vi "Trans_FPGA.vi"() -> ()   [LabVIEW 2016]
uses:
  <vilib>/LabVIEW Targets/FPGA/cRIO/shared/nicrio_ModuleControls/nicrio_cRIO-9871_BaudRateEnum.ctl
  <vilib>/LabVIEW Targets/FPGA/cRIO/shared/nicrio_ModuleControls/nicrio_cRIO-9871_ParityEnum.ctl
  <vilib>/LabVIEW Targets/FPGA/cRIO/shared/nicrio_ModuleControls/nicrio_cRIO-9871_StopBitsEnum.ctl
  <vilib>/LabVIEW Targets/FPGA/cRIO/shared/nicrio_ModuleControls/nicrio_cRIO-9871_DataBitsEnum.ctl
  <vilib>/Platform/TimedLoop/XDataNode/timing_clust.ctl
  <vilib>/Platform/TimedLoop/XDataNode/nitl_modes.ctl
  <vilib>/Platform/TimedLoop/XDataNode/wakeup.ctl
  <vilib>/rvi/FXPMathLib/basic elements/FxpIntAccumulator/subVIs/nifxpmath_IntAccumulator_SimConfig.ctl
  <vilib>/rvi/Emulation/niFpgaGetClockAttributes.vi
  <vilib>/rvi/Emulation/niFpgaSctlEmulationGetInTimedLoop.vi
  <vilib>/rvi/Emulation/niFpgaEmulationReportErrorSimple.vi
  <vilib>/rvi/eio/common/nirviEmuTemplateMethod_errors.vi
  <vilib>/rvi/Emulation/niFpgaCriticalErrorInLSC.vi
  <vilib>/rvi/Analysis/common/codeGenErrors/XNode/niFpgaXNodeCodeGenErrorHandle.vi
  <vilib>/rvi/FXPMathLib/basic elements/FxpIntAccumulator/simVIs/DllFxpIntAccumulator_sub.vi
  <vilib>/rvi/eio/common/nirviEmuTemplatePropertySet_errors.vi
  <vilib>/eio/EIONode/EIONode.xnode
  <vilib>/rvi/Analysis/measure/dc-rms/XNode/niFpgaDC-RMS.xnode
  <vilib>/Platform/TimedLoop/XDataNode/XDataNode.xnode
  <vilib>/rvi/FXPMathLib/basic elements/FxpIntAccumulator/XNode/nifxpmath_IntAccumulator.xnode
  <vilib>/rvi/FXPMathLib/FxpMul/XNode/nifxpmath_Multiplier.xnode
  <vilib>/eio/EIOPropertyNode/EIOPropertyNode.xnode
  <vilib>/eio/EIOMethodNode/EIOMethodNode.xnode
  <vilib>/Platform/TimedLoop/XDataNode/XDNodeRunTimeDep.lvlib
  <vilib>/rvi/FXPMathLib/sim/FxpSim.dll
  <vilib>/rvi/eio/common/nirviEmuTemplatePropertyGet_errors.vi
  <vilib>/rvi/eio/common/nirviEmuTemplatePropertyGet_noerrors.vi
  <vilib>/rvi/eio/common/nirviEmuTemplatePropertySet_noerrors.vi
panel:
  in  "Y-steerer+ V set":fxp<+/-,20,5>
  in  "Y-steerer- V set":fxp<+/-,20,5>
  in  "ExB+ V set":fxp<+/-,20,5>
  in  "ExB- V set":fxp<+/-,20,5>
  in  "X-steerer- V set":fxp<+/-,20,5>
  in  "X-steerer+ V set":fxp<+/-,20,5>
  out "ExB- I read":fxp<+/-,26,5>
  out "ExB- V read":fxp<+/-,26,5>
  out "ExB+ I read":fxp<+/-,26,5>
  out "ExB+ V read":fxp<+/-,26,5>
  out "Y-steerer- I read":fxp<+/-,26,5>
  out "Y-steerer- V read":fxp<+/-,26,5>
  out "Y-steerer+ I read":fxp<+/-,26,5>
  out "Y-steerer+ V read":fxp<+/-,26,5>
  out "X-steerer- I read":fxp<+/-,26,5>
  out "X-steerer- V read":fxp<+/-,26,5>
  out "X-steerer+ I read":fxp<+/-,26,5>
  out "X-steerer+ V read":fxp<+/-,26,5>
  in  "switch mag ps trig":u8[](array[numeric])=[0, 0, 0]
  in  "Switch Mag addr":u8[](array[numeric])=[0, 0, 0, 0, 0, 0, 0, 0]
  out "Switch Object Vacuum Error":errorcluster
  out "Analyze Image Vacuum Error":errorcluster
  out "Switch PS error":errorcluster
  out "ExB PS error":errorcluster
  out "Analyzer PS error":errorcluster
  out "9264 error":errorcluster
  out "9205 error":errorcluster
  in  "RT error":bool
  in  "switch mag ps set":u8[](array[numeric])=[0, 0, 0, 0, 0, 0, 0, 0, 0, 0, 0]
  out "Switch mag data":u8
  out "Switch Mag Hall Probe Timed out":bool
  out "switch mag field":u8[](array[numeric])
  out "Switch Hall Probe error":errorcluster
  in  "trans ExB mag ps set":u8[](array[numeric])=[0, 0, 0, 0, 0, 0, 0, 0, 0, 0]
  in  "analyzer mag ps set":u8[](array[numeric])=[0, 0, 0, 0, 0, 0, 0, 0, 0, 0]
  out "analyzer mag data":u8
  out "Timed Out":bool
  out "analyzer mag field":u8[](array[numeric])
  out "Analyzer Hall Probe error":errorcluster
  out "Ion gauge 4":u8[](array[numeric])
  out "Convectron 4":u8[](array[numeric])
  out "Convectron 3":u8[](array[numeric])
  out "Ion gauge 3":u8[](array[numeric])
  out "Ion gauge 2":u8[](array[numeric])
  out "Convectron 2":u8[](array[numeric])
  out "Convectron 1":u8[](array[numeric])
  out "Ion gauge 1":u8[](array[numeric])
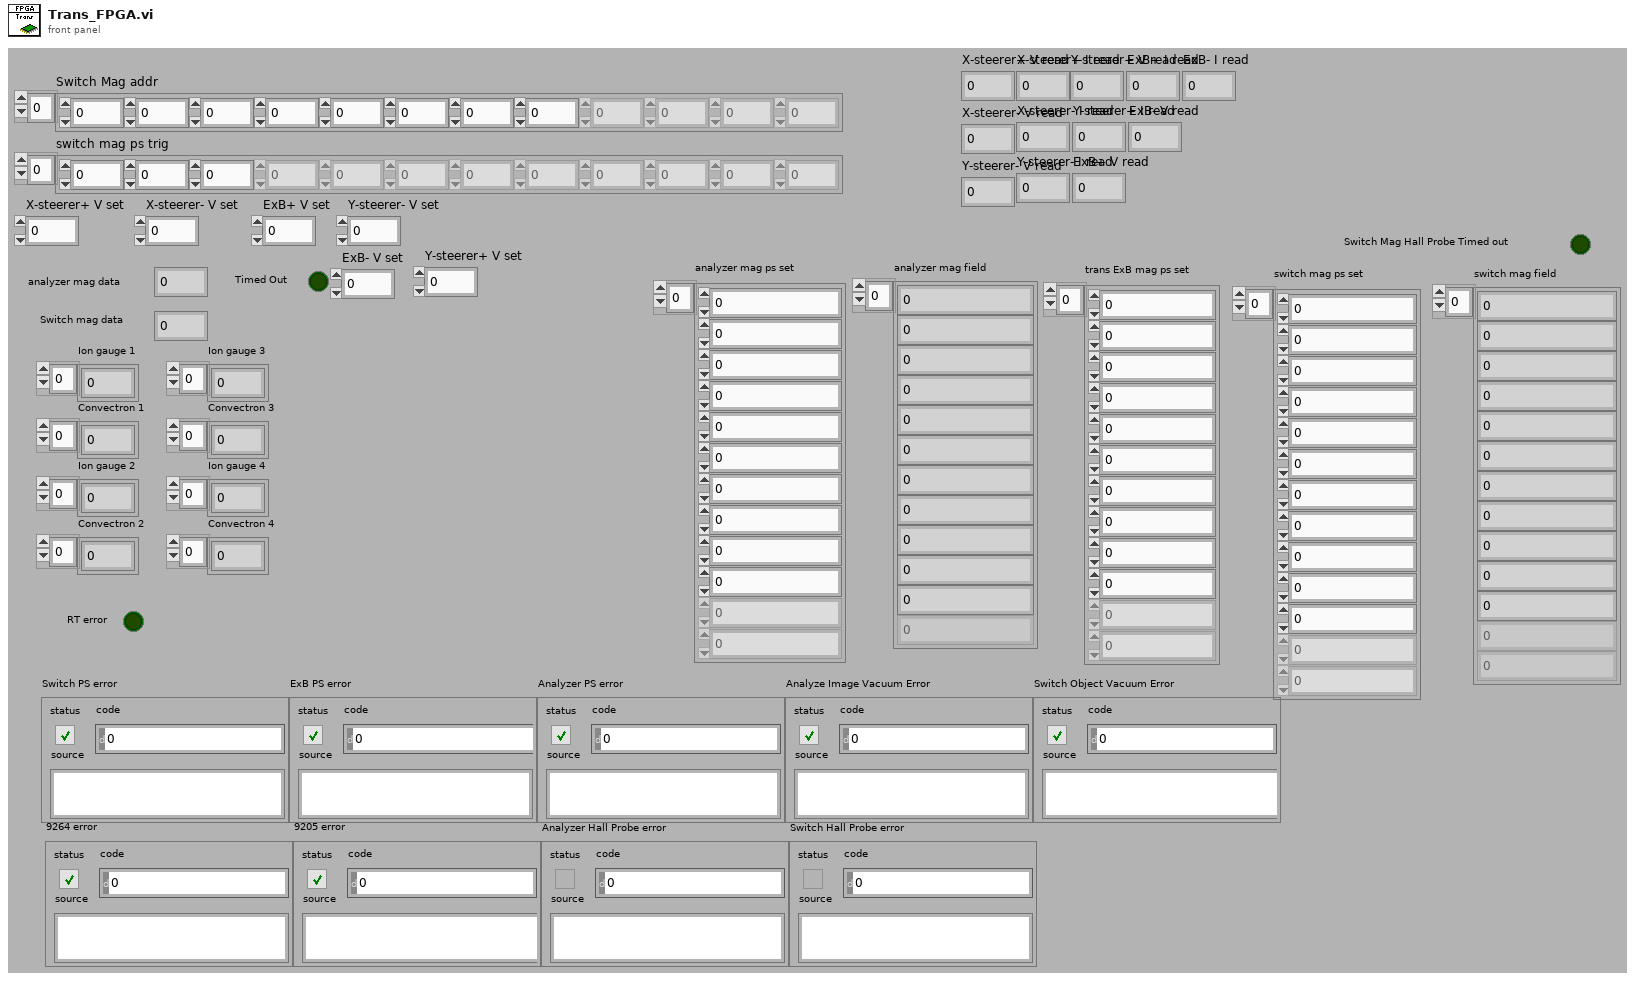
[diagram p1: front panel]
types:
  T1 = typedef "nicrio_cRIO-9871_BaudRateEnum.ctl" = enum16{"75 bps", "110 bps", "134 bps", "150 bps", "300 bps", "600 bps", "1200 bps", "1800 bps", "2400 bps", "4800 bps", "7200 bps", "9600 bps", "14.4 kbps", "19.2 kbps", "28.8 kbps", "38.4 kbps", "57.6 kbps", "115.2 kbps", "230.4 kbps", "460.8 kbps", "921.6 kbps"}
  T2 = typedef "nicrio_cRIO-9871_DataBitsEnum.ctl" = enum8{"5", "6", "7", "8"}
  T3 = typedef "nicrio_cRIO-9871_StopBitsEnum.ctl" = enum8{"1", "1.5", "2"}
  T4 = typedef "nicrio_cRIO-9871_ParityEnum.ctl" = enum8{"None", "Odd", "Even", "Mark", "Space"}
  T5 = typedef "XDNodeRunTimeDep.lvlib/timing_clust.ctl" = cluster{"Expected End [f-1]":u64, "Actual End [f-1]":u64, "Finished Late? [f-1]":bool, "Expected End [i-1]":u64, "Actual End [i-1]":u64, "Finished Late? [i-1]":bool, "Expected Start [i]":u64, "Actual Start [i]":u64, "Expected Start [f]":u64, "Actual Start [f]":u64, "Source Name":string, "Structure Name":string, "Period":i64, "Deadline":i64, "Offset":i64, "Start":i64, "Priority":i32, "Timeout":i32, "Mode":T6, "Wakeup Reason":T7, "Error":errorcluster, "Source Type":string, "Secondary Source Type":string, "Global End Time":u64, "Global Start Time":u64, "Frame Duration":u64, "Iteration Duration":u64, "Assigned CPU":i32, "I/O Scan Engine Mode":u32}
  T6 = typedef "XDNodeRunTimeDep.lvlib/nitl_modes.ctl" = enum32{"No Change", "Process missed periods, maintain original phase", "Discard missed periods, maintain original phase", "Process missed periods, ignore original phase", "Discard missed periods, ignore original phase"}
  T7 = typedef "XDNodeRunTimeDep.lvlib/wakeup.ctl" = enum32{"Normal", "Aborted", "Asynchronous wakeup", "Timing source error", "Timed loop error", "Timeout"}
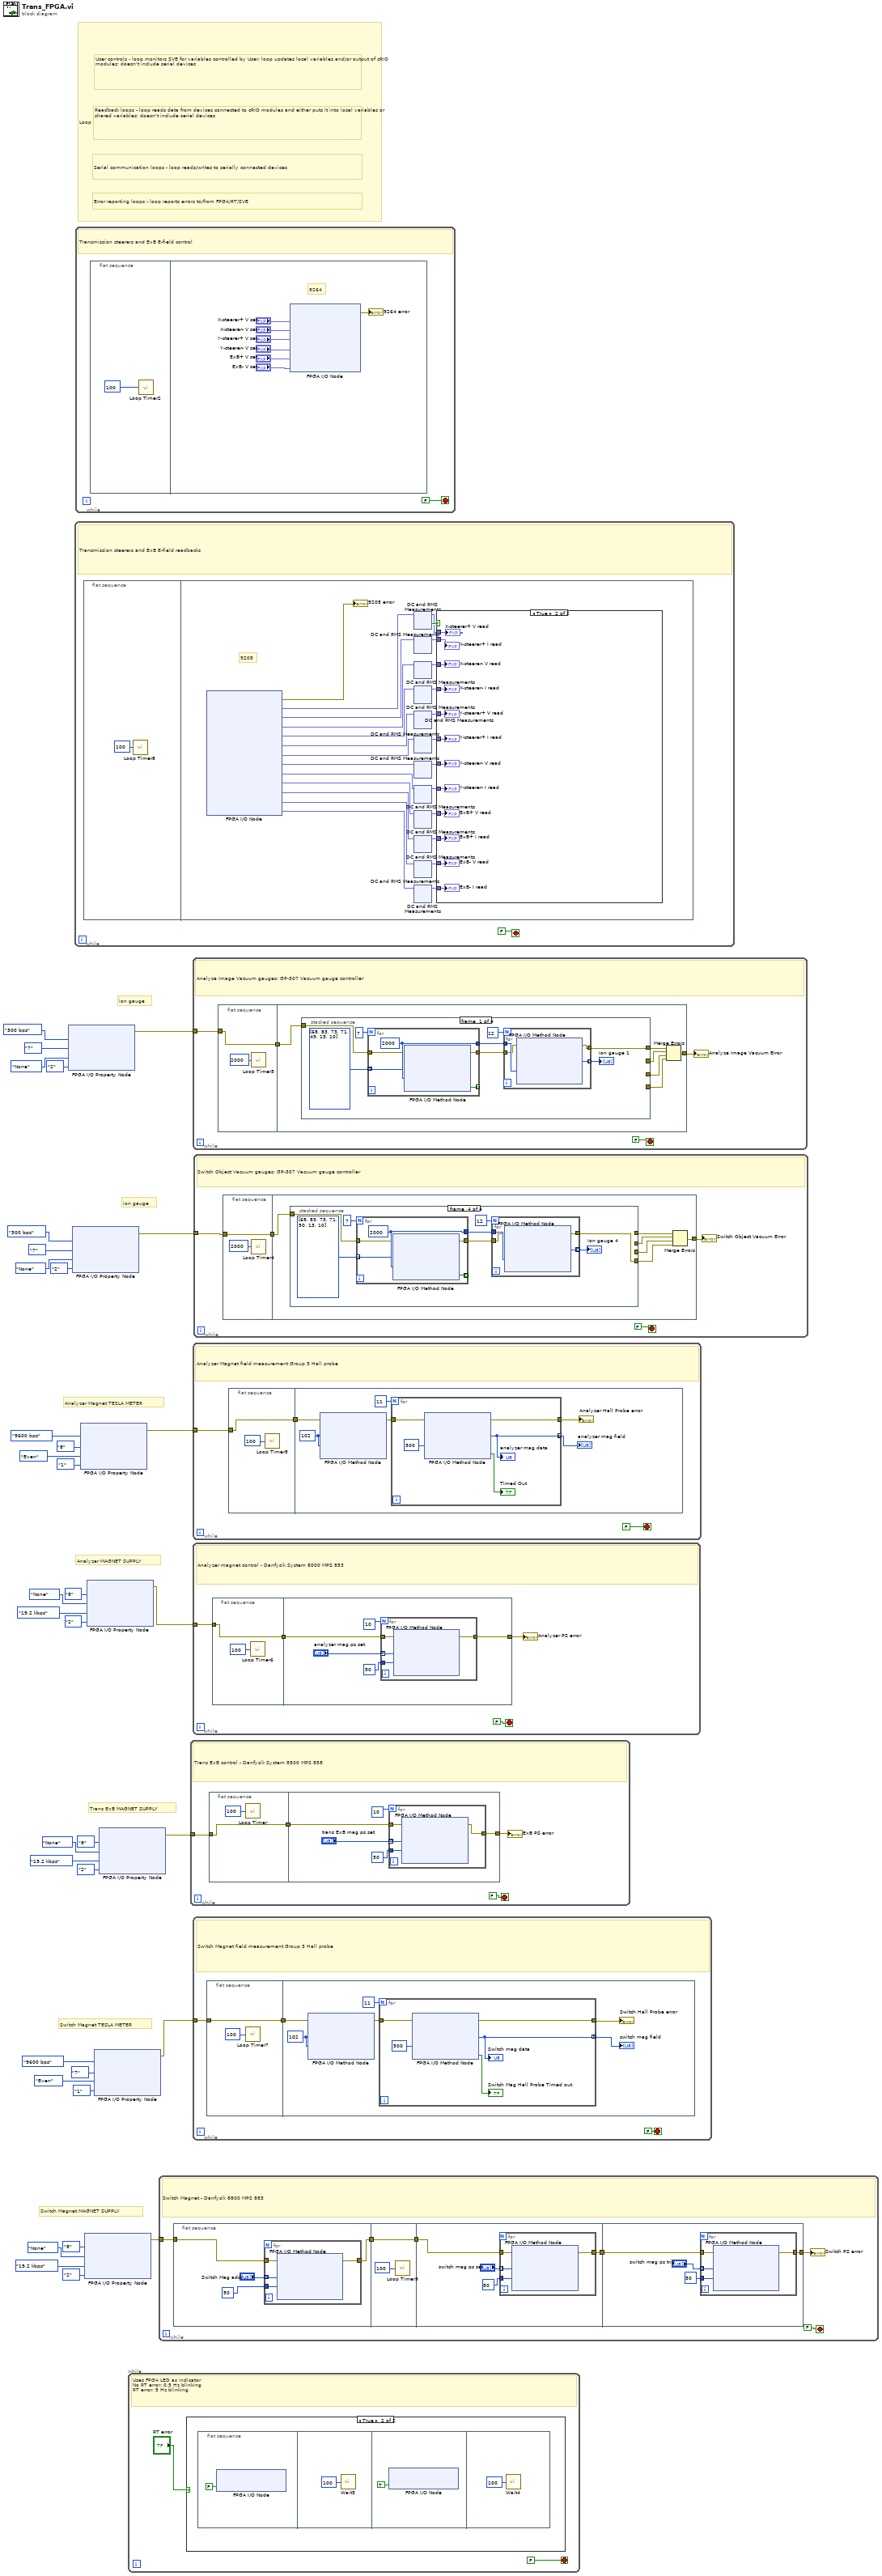
[diagram p0: block diagram]
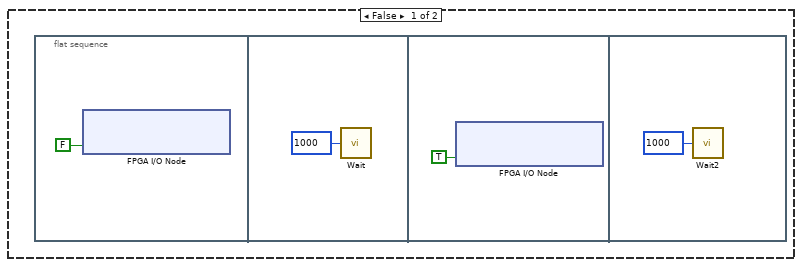
[diagram p2: hidden frame]
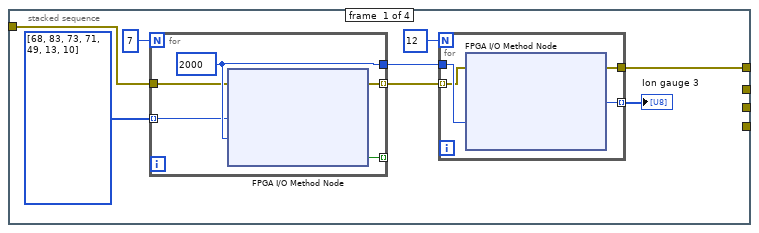
[diagram p4: hidden frame]
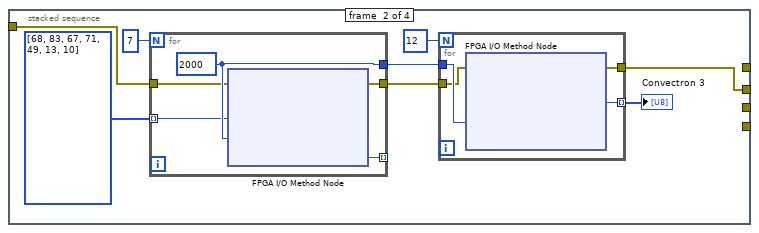
[diagram p5: hidden frame]
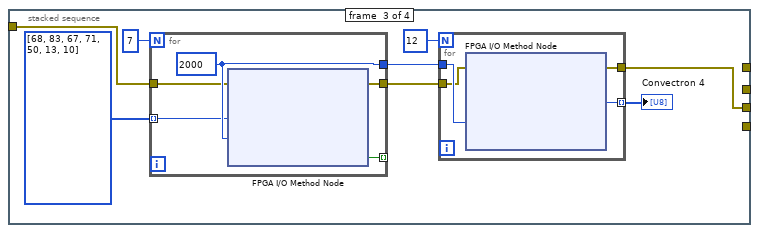
[diagram p6: hidden frame]
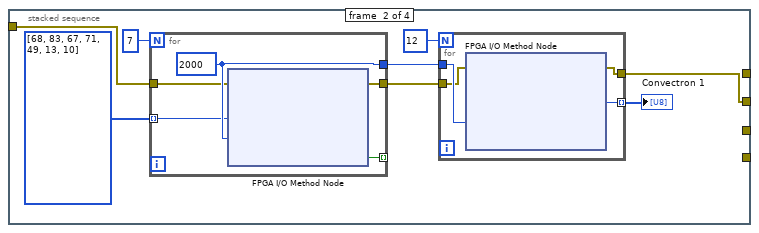
[diagram p7: hidden frame]
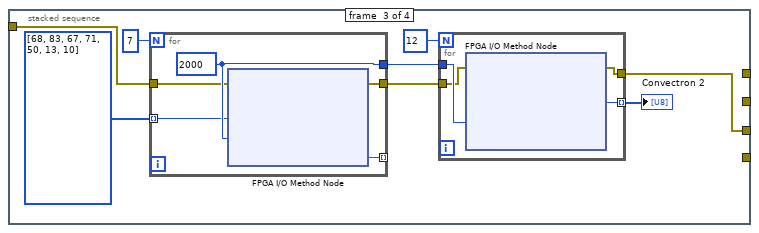
[diagram p8: hidden frame]
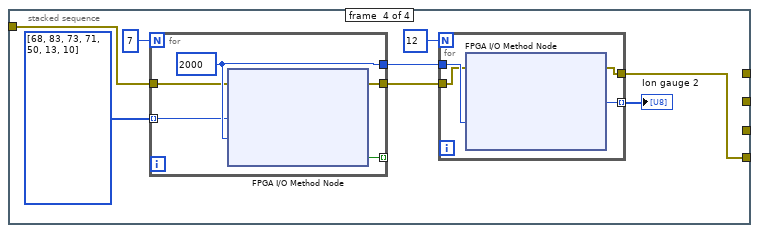
[diagram p9: hidden frame]
diagram:
  # "Error reporting loops - loop reports errors to/from FPGA/RT/SVE"
  # "Serial communication loops - loop reads/writes to serially connected devices"
  # "Readback loops - loop reads data from devices connected to cRIO modules and either puts it into local variables or shared variables; doesn't include serial devices"
  # "User controls - loop monitors SVE for variables controlled by User; loop updates local variables and/or output of cRIO modules; doesn't include serial devices"
  # "Loop legend - loops are color coded by responsibility"
  # "Switch Magnet TESLA METER"
  # "Switch Magnet MAGNET SUPPLY"
  # "Trans ExB MAGNET SUPPLY"
  # "ion gauge"
  # "Analyzer MAGNET SUPPLY"
  # "Analyzer Magnet TESLA METER"
  # "ion gauge"
  n1 = xnode "FPGA I/O Property Node"("Baud Rate"=nicrio_cRIO-9871_BaudRateEnum."300 bps", "Data Bits"=nicrio_cRIO-9871_DataBitsEnum."7", "Parity"=nicrio_cRIO-9871_ParityEnum."None", "Stop Bits"=nicrio_cRIO-9871_StopBitsEnum."2") -> ("error out"=w6:errorcluster)  [unwired: 2 in, 1 out]
  n2 = xnode "FPGA I/O Property Node"("Baud Rate"=nicrio_cRIO-9871_BaudRateEnum."300 bps", "Data Bits"=nicrio_cRIO-9871_DataBitsEnum."7", "Parity"=nicrio_cRIO-9871_ParityEnum."None", "Stop Bits"=nicrio_cRIO-9871_StopBitsEnum."2") -> ("error out"=w7:errorcluster)  [unwired: 2 in, 1 out]
  n3 = while {
    stop <- FALSE stop-if-true
    # "Transmission steerers and ExB E-field readbacks"
    n4 = flat-sequence {
      frame #0 {
        n5 = call "Loop Timer8"("Count(uSec)"=u32 100 ("Count(Ticks)")) -> ()  [unwired: 1 out]
      }
      frame #1 {
        # "9205"
        n6 = xnode "FPGA I/O Node"() -> ("error out"=→"9205 error":errorcluster, "X-steerer+ V read"=w62:fxp<+/-,26,5>, "X-steerer+ I read"=w60:fxp<+/-,26,5>, "X-steerer- V read"=w58:fxp<+/-,26,5>, "X-steerer- I read"=w56:fxp<+/-,26,5>, "Y-steerer+ V read"=w54:fxp<+/-,26,5>, "Y-steerer+ I read"=w52:fxp<+/-,26,5>, "Y-steerer- V read"=w50:fxp<+/-,26,5>, "Y-steerer- I read"=w48:fxp<+/-,26,5>, "ExB+ V read"=w46:fxp<+/-,26,5>, "ExB+ I read"=w44:fxp<+/-,26,5>, "ExB- V read"=w42:fxp<+/-,26,5>, "ExB- I read"=w40:fxp<+/-,26,5>)  [unwired: 13 in, 12 out]
        n7 = xnode "DC and RMS Measurements"("input data"=w62) -> ("DC"=w61:fxp<+/-,26,5>, "output valid"=w63:bool)  [unwired: 1 in]
        n8 = xnode "DC and RMS Measurements"("input data"=w60) -> ("DC"=w59:fxp<+/-,26,5>)  [unwired: 1 in, 1 out]
        n9 = xnode "DC and RMS Measurements"("input data"=w58) -> ("DC"=w57:fxp<+/-,26,5>)  [unwired: 1 in, 1 out]
        n10 = xnode "DC and RMS Measurements"("input data"=w56) -> ("DC"=w55:fxp<+/-,26,5>)  [unwired: 1 in, 1 out]
        n11 = xnode "DC and RMS Measurements"("input data"=w54) -> ("DC"=w53:fxp<+/-,26,5>)  [unwired: 1 in, 1 out]
        n12 = xnode "DC and RMS Measurements"("input data"=w52) -> ("DC"=w51:fxp<+/-,26,5>)  [unwired: 1 in, 1 out]
        n13 = xnode "DC and RMS Measurements"("input data"=w50) -> ("DC"=w49:fxp<+/-,26,5>)  [unwired: 1 in, 1 out]
        n14 = xnode "DC and RMS Measurements"("input data"=w48) -> ("DC"=w47:fxp<+/-,26,5>)  [unwired: 1 in, 1 out]
        n15 = xnode "DC and RMS Measurements"("input data"=w46) -> ("DC"=w45:fxp<+/-,26,5>)  [unwired: 1 in, 1 out]
        n16 = xnode "DC and RMS Measurements"("input data"=w44) -> ("DC"=w43:fxp<+/-,26,5>)  [unwired: 1 in, 1 out]
        n17 = xnode "DC and RMS Measurements"("input data"=w42) -> ("DC"=w41:fxp<+/-,26,5>)  [unwired: 1 in, 1 out]
        n18 = xnode "DC and RMS Measurements"("input data"=w40) -> ("DC"=w39:fxp<+/-,26,5>)  [unwired: 1 in, 1 out]
        n19 = case shown="True" w63 {
          tunnel: w61 -> [_ w75]
          tunnel: w59 -> [_ w74]
          tunnel: w57 -> [_ w73]
          tunnel: w55 -> [_ w72]
          tunnel: w53 -> [_ w71]
          tunnel: w51 -> [_ w70]
          tunnel: w49 -> [_ w69]
          tunnel: w47 -> [_ w68]
          tunnel: w45 -> [_ w67]
          tunnel: w43 -> [_ w66]
          tunnel: w41 -> [_ w65]
          tunnel: w39 -> [_ w64]
          frame False {
          }
          frame True {
            "X-steerer+ V read" <- w75
            "X-steerer+ I read" <- w74
            "X-steerer- V read" <- w73
            "X-steerer- I read" <- w72
            "Y-steerer+ V read" <- w71
            "Y-steerer+ I read" <- w70
            "Y-steerer- V read" <- w69
            "Y-steerer- I read" <- w68
            "ExB+ V read" <- w67
            "ExB+ I read" <- w66
            "ExB- V read" <- w65
            "ExB- I read" <- w64
          }
        }
      }
    }
  }
  n20 = while {
    stop <- FALSE stop-if-true
    # "Transmission steerers and ExB E-field control"
    n21 = flat-sequence {
      frame #0 {
        n22 = call "Loop Timer2"("Count(mSec)"=u32 100 ("Count(Ticks)")) -> ()  [unwired: 1 out]
      }
      frame #1 {
        # "9264"
        n23 = xnode "FPGA I/O Node"("X-steerer+ V set"="X-steerer+ V set", "X-steerer- V set"="X-steerer- V set", "Y-steerer+ V set"="Y-steerer+ V set", "Y-steerer- V set"="Y-steerer- V set", "ExB+ V set"="ExB+ V set", "ExB- V set"="ExB- V set") -> ("error out"=→"9264 error":errorcluster)  [unwired: 7 in, 6 out]
      }
    }
  }
  n24 = xnode "FPGA I/O Property Node"("Baud Rate"=nicrio_cRIO-9871_BaudRateEnum."9600 bps", "Data Bits"=nicrio_cRIO-9871_DataBitsEnum."8", "Parity"=nicrio_cRIO-9871_ParityEnum."Even", "Stop Bits"=nicrio_cRIO-9871_StopBitsEnum."1") -> ("error out"=w8:errorcluster)  [unwired: 2 in, 1 out]
  n25 = xnode "FPGA I/O Property Node"("Data Bits"=nicrio_cRIO-9871_DataBitsEnum."8", "Parity"=nicrio_cRIO-9871_ParityEnum."None", "Baud Rate"=nicrio_cRIO-9871_BaudRateEnum."19.2 kbps", "Stop Bits"=nicrio_cRIO-9871_StopBitsEnum."2") -> ("error out"=w10:errorcluster)  [unwired: 2 in, 1 out]
  n26 = xnode "FPGA I/O Property Node"("Data Bits"=nicrio_cRIO-9871_DataBitsEnum."8", "Parity"=nicrio_cRIO-9871_ParityEnum."None", "Baud Rate"=nicrio_cRIO-9871_BaudRateEnum."19.2 kbps", "Stop Bits"=nicrio_cRIO-9871_StopBitsEnum."2") -> ("error out"=w9:errorcluster)  [unwired: 2 in, 1 out]
  n27 = xnode "FPGA I/O Property Node"("Baud Rate"=nicrio_cRIO-9871_BaudRateEnum."9600 bps", "Data Bits"=nicrio_cRIO-9871_DataBitsEnum."7", "Parity"=nicrio_cRIO-9871_ParityEnum."Even", "Stop Bits"=nicrio_cRIO-9871_StopBitsEnum."1") -> ("error out"=w11:errorcluster)  [unwired: 2 in, 1 out]
  n28 = xnode "FPGA I/O Property Node"("Data Bits"=nicrio_cRIO-9871_DataBitsEnum."8", "Parity"=nicrio_cRIO-9871_ParityEnum."None", "Baud Rate"=nicrio_cRIO-9871_BaudRateEnum."19.2 kbps", "Stop Bits"=nicrio_cRIO-9871_StopBitsEnum."2") -> ("error out"=w12:errorcluster)  [unwired: 2 in, 1 out]
  n29 = while {
    stop <- FALSE stop-if-true
    # "Uses FPGA LED as indicator\nNo RT error: 0.5 Hz blinking\nRT error: 5 Hz blinking"
    n30 = case shown="True" "RT error" {
      frame False {
        n31 = flat-sequence {
          frame #0 {
            n32 = xnode "FPGA I/O Node"("USER FPGA LED"=FALSE ("FPGA LED")) -> ()  [unwired: 1 in, 1 out]
          }
          frame #1 {
            n33 = call "Wait"("Count(mSec)"=u16 1000) -> ()  [unwired: 1 out]
          }
          frame #2 {
            n34 = xnode "FPGA I/O Node"("USER FPGA LED"=TRUE ("FPGA LED")) -> ()  [unwired: 1 in, 1 out]
          }
          frame #3 {
            n35 = call "Wait2"("Count(mSec)"=u16 1000) -> ()  [unwired: 1 out]
          }
        }
      }
      frame True {
        n36 = flat-sequence {
          frame #0 {
            n37 = xnode "FPGA I/O Node"("USER FPGA LED"=FALSE ("FPGA LED")) -> ()  [unwired: 1 in, 1 out]
          }
          frame #1 {
            n38 = call "Wait3"("Count(mSec)"=u16 100) -> ()  [unwired: 1 out]
          }
          frame #2 {
            n39 = xnode "FPGA I/O Node"("USER FPGA LED"=TRUE ("FPGA LED")) -> ()  [unwired: 1 in, 1 out]
          }
          frame #3 {
            n40 = call "Wait4"("Count(mSec)"=u16 100) -> ()  [unwired: 1 out]
          }
        }
      }
    }
  }
  n41 = while {
    tunnel: w10 -> [w1057]
    stop <- FALSE stop-if-true
    # "Switch Magnet - Danfysik 8800 MPS 883"
    n42 = flat-sequence {
      tunnel: w1057 -> [w1063]
      tunnel: [w1062] -> w1056
      tunnel: [w1069] -> w1058
      tunnel: w1056 -> [w1069]
      tunnel: w1058 -> [w1071]
      tunnel: [w1072] -> w1055
      tunnel: [w1082] -> w1059
      tunnel: w1055 -> [w1081]
      frame #0 {
        n43 = for {
          tunnel: 50 ("Timeout (ms)") -> [w1068]
          tunnel: "Switch Mag addr" -> [w1067] mode=indexing
          tunnel: [w1066] -> w1062
          tunnel: w1063 -> [w1065]
          n44 = xnode "FPGA I/O Method Node"("error in"=w1065, "Data"=w1067, "Timeout (ms)"=w1068) -> ("error out"=w1066:errorcluster)  [unwired: 1 in, 2 out]
        }
      }
      frame #1 {
        n45 = call "Loop Timer9"("Count(mSec)"=u32 100) -> ()  [unwired: 1 out]
      }
      frame #2 {
        n46 = for {
          tunnel: 50 ("Timeout (ms)") -> [w1078]
          tunnel: "switch mag ps set" -> [w1077] mode=indexing
          tunnel: [w1076] -> w1072
          tunnel: w1071 -> [w1075]
          n47 = xnode "FPGA I/O Method Node"("error in"=w1075, "Data"=w1077, "Timeout (ms)"=w1078) -> ("error out"=w1076:errorcluster)  [unwired: 1 in, 2 out]
        }
      }
      frame #3 {
        n48 = for {
          tunnel: 50 ("Timeout (ms)") -> [w1086]
          tunnel: "switch mag ps trig" -> [w1085] mode=indexing
          tunnel: [w1084] -> w1082
          tunnel: w1081 -> [w1083]
          n49 = xnode "FPGA I/O Method Node"("error in"=w1083, "Data"=w1085, "Timeout (ms)"=w1086) -> ("error out"=w1084:errorcluster)  [unwired: 1 in, 2 out]
        }
      }
    }
    "Switch PS error" <- w1059
  }
  n50 = while {
    tunnel: w12 -> [w1088]
    stop <- FALSE stop-if-true
    # "Trans ExB control - Danfysik System 8500 MPS 858"
    n51 = flat-sequence {
      tunnel: w1088 -> [w1091]
      tunnel: [w1091] -> w1087
      tunnel: [w1094] -> w1089
      tunnel: w1087 -> [w1093]
      frame #0 {
        n52 = call "Loop Timer"("Count(mSec)"=u32 100) -> ()  [unwired: 1 out]
      }
      frame #1 {
        n53 = for {
          N: 10 -> [_]
          tunnel: 50 ("Timeout (ms)") -> [w1101]
          tunnel: "trans ExB mag ps set" -> [w1100] mode=indexing
          tunnel: [w1099] -> w1094
          tunnel: w1093 -> [w1098]
          n54 = xnode "FPGA I/O Method Node"("error in"=w1098, "Data"=w1100, "Timeout (ms)"=w1101) -> ("error out"=w1099:errorcluster)  [unwired: 1 in, 2 out]
        }
      }
    }
    "ExB PS error" <- w1089
  }
  n55 = while {
    tunnel: w6 -> [w1104]
    stop <- FALSE stop-if-true
    # "Analyze Image Vacuum gauges: GP-307 Vacuum gauge controller"
    n56 = flat-sequence {
      tunnel: w1104 -> [w1106]
      tunnel: [w1106] -> w1103
      tunnel: w1103 -> [w1113]
      tunnel: [w1111] -> w1102
      frame #0 {
        n57 = call "Loop Timer3"("Count(mSec)"=u32 2000 ("Count(Ticks)")) -> ()  [unwired: 1 out]
      }
      frame #1 {
        n58 = stacked-sequence {
          tunnel: w1113 -> [w1116 w1133 w1150 w1166]
          tunnel: [w1114 _ _ _] -> w1112
          tunnel: [_ w1131 _ _] -> w1110
          tunnel: [_ _ w1148 _] -> w1109
          tunnel: [_ _ _ w1165] -> w1108
          frame #0 {
            n59 = for {
              N: 7 -> [_]
              tunnel: [w1130] -> w1121
              tunnel: [w1129] -> _ mode=indexing
              tunnel: u8[] [68, 83, 73, 71, 49, 13, 10] ("unsigned byte array") -> [w1128] mode=indexing
              tunnel: w1116 -> [w1127]
              tunnel: [w1126] -> w1115
              w1130 = 2000 ("Timeout (ms)")
              n60 = xnode "FPGA I/O Method Node"("error in"=w1127, "Data"=w1128, "Timeout (ms)"=w1130) -> ("error out"=w1126:errorcluster, "Timed Out"=w1129:bool)  [unwired: 1 in, 1 out]
            }
            n61 = for {
              N: 12 -> [_]
              tunnel: w1121 -> [w1125]
              tunnel: [w1124] -> w1117 mode=indexing
              tunnel: w1115 -> [w1123]
              tunnel: [w1122] -> w1114
              n62 = xnode "FPGA I/O Method Node"("error in"=w1123, "Timeout (ms)"=w1125) -> ("error out"=w1122:errorcluster, "Data"=w1124:u8)  [unwired: 1 in, 2 out]
            }
            "Ion gauge 1" <- w1117
          }
          frame #1 {
            n63 = for {
              N: 7 -> [_]
              tunnel: [w1147] -> w1138
              tunnel: [w1146] -> _ mode=indexing
              tunnel: u8[] [68, 83, 67, 71, 49, 13, 10] ("unsigned byte array") -> [w1145] mode=indexing
              tunnel: w1133 -> [w1144]
              tunnel: [w1143] -> w1132
              w1147 = 2000 ("Timeout (ms)")
              n64 = xnode "FPGA I/O Method Node"("error in"=w1144, "Data"=w1145, "Timeout (ms)"=w1147) -> ("error out"=w1143:errorcluster, "Timed Out"=w1146:bool)  [unwired: 1 in, 1 out]
            }
            n65 = for {
              N: 12 -> [_]
              tunnel: w1138 -> [w1142]
              tunnel: [w1141] -> w1134 mode=indexing
              tunnel: w1132 -> [w1140]
              tunnel: [w1139] -> w1131
              n66 = xnode "FPGA I/O Method Node"("error in"=w1140, "Timeout (ms)"=w1142) -> ("error out"=w1139:errorcluster, "Data"=w1141:u8)  [unwired: 1 in, 2 out]
            }
            "Convectron 1" <- w1134
          }
          frame #2 {
            n67 = for {
              N: 7 -> [_]
              tunnel: [w1164] -> w1155
              tunnel: [w1163] -> _ mode=indexing
              tunnel: u8[] [68, 83, 67, 71, 50, 13, 10] ("unsigned byte array") -> [w1162] mode=indexing
              tunnel: w1150 -> [w1161]
              tunnel: [w1160] -> w1149
              w1164 = 2000 ("Timeout (ms)")
              n68 = xnode "FPGA I/O Method Node"("error in"=w1161, "Data"=w1162, "Timeout (ms)"=w1164) -> ("error out"=w1160:errorcluster, "Timed Out"=w1163:bool)  [unwired: 1 in, 1 out]
            }
            n69 = for {
              N: 12 -> [_]
              tunnel: w1155 -> [w1159]
              tunnel: [w1158] -> w1151 mode=indexing
              tunnel: w1149 -> [w1157]
              tunnel: [w1156] -> w1148
              n70 = xnode "FPGA I/O Method Node"("error in"=w1157, "Timeout (ms)"=w1159) -> ("error out"=w1156:errorcluster, "Data"=w1158:u8)  [unwired: 1 in, 2 out]
            }
            "Convectron 2" <- w1151
          }
          frame #3 {
            n71 = for {
              N: 7 -> [_]
              tunnel: [w1181] -> w1172
              tunnel: [w1180] -> _ mode=indexing
              tunnel: u8[] [68, 83, 73, 71, 50, 13, 10] ("unsigned byte array") -> [w1179] mode=indexing
              tunnel: [w1178] -> w1167
              tunnel: w1166 -> [w1177]
              w1181 = 2000 ("Timeout (ms)")
              n72 = xnode "FPGA I/O Method Node"("error in"=w1177, "Data"=w1179, "Timeout (ms)"=w1181) -> ("error out"=w1178:errorcluster, "Timed Out"=w1180:bool)  [unwired: 1 in, 1 out]
            }
            n73 = for {
              N: 12 -> [_]
              tunnel: w1172 -> [w1176]
              tunnel: [w1175] -> w1168 mode=indexing
              tunnel: w1167 -> [w1174]
              tunnel: [w1173] -> w1165
              n74 = xnode "FPGA I/O Method Node"("error in"=w1174, "Timeout (ms)"=w1176) -> ("error out"=w1173:errorcluster, "Data"=w1175:u8)  [unwired: 1 in, 2 out]
            }
            "Ion gauge 2" <- w1168
          }
        }
        n75 = Merge Errors(w1112, w1110, w1109, w1108) -> (w1111:errorcluster)
      }
    }
    "Analyze Image Vacuum Error" <- w1102
  }
  n76 = while {
    tunnel: w8 -> [w1183]
    stop <- FALSE stop-if-true
    # "Analyzer Magnet field measurement Group 3 Hall probe"
    n77 = flat-sequence {
      tunnel: w1183 -> [w1185]
      tunnel: [w1185] -> w1182
      tunnel: w1182 -> [w1187]
      frame #0 {
        n78 = call "Loop Timer5"("Count(mSec)"=u32 100) -> ()  [unwired: 1 out]
      }
      frame #1 {
        w1191 = u8 102 ("Data")
        n79 = xnode "FPGA I/O Method Node"("error in"=w1187, "Data"=w1191, "Timeout (ms)"=w1191) -> ("error out"=w1190:errorcluster)  [unwired: 1 in, 2 out]
        n80 = for {
          N: 11 ("Numeric 3") -> [_]
          tunnel: [w1195] -> w1188 mode=indexing
          tunnel: w1190 -> [w1194]
          tunnel: [w1193] -> w1189
          n81 = xnode "FPGA I/O Method Node"("error in"=w1194, "Timeout (ms)"=500) -> ("error out"=w1193:errorcluster, "Data"=w1195:u8, "Timed Out"=→"Timed Out":bool)  [unwired: 1 in, 1 out]
          "analyzer mag data" <- w1195
        }
        "analyzer mag field" <- w1188
        "Analyzer Hall Probe error" <- w1189
      }
    }
  }
  n82 = while {
    tunnel: w9 -> [w1199]
    stop <- FALSE stop-if-true
    # "Analyzer magnet control - Danfysik System 8000 MPS 853"
    n83 = flat-sequence {
      tunnel: w1199 -> [w1202]
      tunnel: [w1202] -> w1198
      tunnel: [w1205] -> w1200
      tunnel: w1198 -> [w1204]
      frame #0 {
        n84 = call "Loop Timer6"("Count(mSec)"=u32 100) -> ()  [unwired: 1 out]
      }
      frame #1 {
        n85 = for {
          N: 10 -> [_]
          tunnel: 50 ("Timeout (ms)") -> [w1212]
          tunnel: "analyzer mag ps set" -> [w1211] mode=indexing
          tunnel: [w1210] -> w1205
          tunnel: w1204 -> [w1209]
          n86 = xnode "FPGA I/O Method Node"("error in"=w1209, "Data"=w1211, "Timeout (ms)"=w1212) -> ("error out"=w1210:errorcluster)  [unwired: 1 in, 2 out]
        }
      }
    }
    "Analyzer PS error" <- w1200
  }
  n87 = while {
    tunnel: w11 -> [w1214]
    stop <- FALSE stop-if-true
    # "Switch Magnet field measurement Group 3 Hall probe"
    n88 = flat-sequence {
      tunnel: w1214 -> [w1216]
      tunnel: [w1216] -> w1213
      tunnel: w1213 -> [w1219]
      frame #0 {
        n89 = call "Loop Timer7"("Count(mSec)"=u32 100) -> ()  [unwired: 1 out]
      }
      frame #1 {
        w1222 = u8 102 ("Data")
        n90 = xnode "FPGA I/O Method Node"("error in"=w1219, "Data"=w1222, "Timeout (ms)"=w1222) -> ("error out"=w1221:errorcluster)  [unwired: 1 in, 2 out]
        n91 = for {
          N: 11 ("Numeric 3") -> [_]
          tunnel: [w1226] -> w1218 mode=indexing
          tunnel: w1221 -> [w1225]
          tunnel: [w1224] -> w1220
          n92 = xnode "FPGA I/O Method Node"("error in"=w1225, "Timeout (ms)"=500) -> ("error out"=w1224:errorcluster, "Data"=w1226:u8, "Timed Out"=→"Switch Mag Hall Probe Timed out":bool)  [unwired: 1 in, 1 out]
          "Switch mag data" <- w1226
        }
        "switch mag field" <- w1218
        "Switch Hall Probe error" <- w1220
      }
    }
  }
  n93 = while {
    tunnel: w7 -> [w1231]
    stop <- FALSE stop-if-true
    # "Switch Object Vacuum gauges: GP-307 Vacuum gauge controller"
    n94 = flat-sequence {
      tunnel: w1231 -> [w1233]
      tunnel: [w1233] -> w1230
      tunnel: w1230 -> [w1240]
      tunnel: [w1238] -> w1229
      frame #0 {
        n95 = call "Loop Timer4"("Count(mSec)"=u32 2000 ("Count(Ticks)")) -> ()  [unwired: 1 out]
      }
      frame #1 {
        n96 = stacked-sequence {
          tunnel: w1240 -> [w1243 w1260 w1277 w1294]
          tunnel: [w1241 _ _ _] -> w1239
          tunnel: [_ w1258 _ _] -> w1237
          tunnel: [_ _ w1275 _] -> w1236
          tunnel: [_ _ _ w1292] -> w1235
          frame #0 {
            n97 = for {
              N: 7 -> [_]
              tunnel: [w1257] -> w1248
              tunnel: [w1256] -> _ mode=indexing
              tunnel: u8[] [68, 83, 73, 71, 49, 13, 10] ("unsigned byte array") -> [w1255] mode=indexing
              tunnel: w1243 -> [w1254]
              tunnel: [w1253] -> w1242 mode=indexing
              w1257 = 2000 ("Timeout (ms)")
              n98 = xnode "FPGA I/O Method Node"("error in"=w1254, "Data"=w1255, "Timeout (ms)"=w1257) -> ("error out"=w1253:errorcluster, "Timed Out"=w1256:bool)  [unwired: 1 in, 1 out]
            }
            n99 = for {
              N: 12 -> [_]
              tunnel: w1248 -> [w1252]
              tunnel: [w1251] -> w1244 mode=indexing
              tunnel: w1242 -> [w1250] mode=indexing
              tunnel: [w1249] -> w1241
              n100 = xnode "FPGA I/O Method Node"("error in"=w1250, "Timeout (ms)"=w1252) -> ("error out"=w1249:errorcluster, "Data"=w1251:u8)  [unwired: 1 in, 2 out]
            }
            "Ion gauge 3" <- w1244
          }
          frame #1 {
            n101 = for {
              N: 7 -> [_]
              tunnel: [w1274] -> w1265
              tunnel: [w1273] -> _ mode=indexing
              tunnel: u8[] [68, 83, 67, 71, 49, 13, 10] ("unsigned byte array") -> [w1272] mode=indexing
              tunnel: w1260 -> [w1271]
              tunnel: [w1270] -> w1259
              w1274 = 2000 ("Timeout (ms)")
              n102 = xnode "FPGA I/O Method Node"("error in"=w1271, "Data"=w1272, "Timeout (ms)"=w1274) -> ("error out"=w1270:errorcluster, "Timed Out"=w1273:bool)  [unwired: 1 in, 1 out]
            }
            n103 = for {
              N: 12 -> [_]
              tunnel: w1265 -> [w1269]
              tunnel: [w1268] -> w1261 mode=indexing
              tunnel: w1259 -> [w1267]
              tunnel: [w1266] -> w1258
              n104 = xnode "FPGA I/O Method Node"("error in"=w1267, "Timeout (ms)"=w1269) -> ("error out"=w1266:errorcluster, "Data"=w1268:u8)  [unwired: 1 in, 2 out]
            }
            "Convectron 3" <- w1261
          }
          frame #2 {
            n105 = for {
              N: 7 -> [_]
              tunnel: [w1291] -> w1282
              tunnel: [w1290] -> _ mode=indexing
              tunnel: u8[] [68, 83, 67, 71, 50, 13, 10] ("unsigned byte array") -> [w1289] mode=indexing
              tunnel: w1277 -> [w1288]
              tunnel: [w1287] -> w1276
              w1291 = 2000 ("Timeout (ms)")
              n106 = xnode "FPGA I/O Method Node"("error in"=w1288, "Data"=w1289, "Timeout (ms)"=w1291) -> ("error out"=w1287:errorcluster, "Timed Out"=w1290:bool)  [unwired: 1 in, 1 out]
            }
            n107 = for {
              N: 12 -> [_]
              tunnel: w1282 -> [w1286]
              tunnel: [w1285] -> w1278 mode=indexing
              tunnel: w1276 -> [w1284]
              tunnel: [w1283] -> w1275
              n108 = xnode "FPGA I/O Method Node"("error in"=w1284, "Timeout (ms)"=w1286) -> ("error out"=w1283:errorcluster, "Data"=w1285:u8)  [unwired: 1 in, 2 out]
            }
            "Convectron 4" <- w1278
          }
          frame #3 {
            n109 = for {
              N: 7 -> [_]
              tunnel: [w1308] -> w1299
              tunnel: [w1307] -> _ mode=indexing
              tunnel: u8[] [68, 83, 73, 71, 50, 13, 10] ("unsigned byte array") -> [w1306] mode=indexing
              tunnel: w1294 -> [w1305]
              tunnel: [w1304] -> w1293
              w1308 = 2000 ("Timeout (ms)")
              n110 = xnode "FPGA I/O Method Node"("error in"=w1305, "Data"=w1306, "Timeout (ms)"=w1308) -> ("error out"=w1304:errorcluster, "Timed Out"=w1307:bool)  [unwired: 1 in, 1 out]
            }
            n111 = for {
              N: 12 -> [_]
              tunnel: w1299 -> [w1303]
              tunnel: [w1302] -> w1295 mode=indexing
              tunnel: w1293 -> [w1301]
              tunnel: [w1300] -> w1292
              n112 = xnode "FPGA I/O Method Node"("error in"=w1301, "Timeout (ms)"=w1303) -> ("error out"=w1300:errorcluster, "Data"=w1302:u8)  [unwired: 1 in, 2 out]
            }
            "Ion gauge 4" <- w1295
          }
        }
        n113 = Merge Errors(w1239, w1237, w1236, w1235) -> (w1238:errorcluster)
      }
    }
    "Switch Object Vacuum Error" <- w1229
  }
